vi "Update FP.vi"(6 "subpanel to main command event":T2, 7 "defer fp updates (T)":bool=TRUE, 8 "error in (no error)":errorcluster, 10 "fp refs":T1, 11 "steering frame ref in":refnum<data-value>) -> (0 "error out":errorcluster, 3 "steering frame ref out":refnum<data-value>)   [LabVIEW 2017, in "NI_Robotics_Configure Steering Frame.lvlib" / "Differential Frame Subpanel.lvlib"]
uses:
  <vilib>/robotics/Dialog/Configure Steering Frame/Differential Frame Subpanel/Differential Frame Subpanel.lvlib
  <vilib>/robotics/Steering/Differential Steering Frame/NI_Robotics_Differential Steering Frame.lvclass
  c:/Program Files (x86)/National Instruments/LabVIEW 2017/vi.lib/robotics/Steering/Steering Frame/NI_Robotics_Steering Frame.lvclass
  <vilib>/robotics/Dialog/Configure Steering Frame/Subpanel to Main Command Event.ctl
  <vilib>/robotics/Dialog/Configure Steering Frame/Subpanel to Main Command.ctl
  <vilib>/robotics/Dialog/Configure Steering Frame/Differential Frame Subpanel/FP Refs.ctl
  <vilib>/robotics/Steering/Differential Steering Frame/NI_Robotics_Differential Steering Frame.lvclass/NI_Robotics_Differential Steering Frame.ctl
  <vilib>/robotics/Steering/Steering Frame/NI_Robotics_Steering Frame.lvclass/NI_Robotics_Steering Frame.ctl
  <vilib>/robotics/Steering/Steering Frame/Get Single Wheel in Steering Frame.vi
  <vilib>/robotics/Steering/Steering Frame/Get Multiple Wheels in Steering Frame.vi
  <vilib>/robotics/Steering/Wheel/Get Fixed Wheel Information.vi
  <vilib>/robotics/Steering/Wheel/NI_Robotics_Wheel.lvclass
  <vilib>/robotics/Steering/Steering Frame/NI_Robotics_Steering Frame.lvclass
  c:/Program Files (x86)/National Instruments/LabVIEW 2017/vi.lib/robotics/Steering/Special Steering Frame/NI_Robotics_Special Steering Frame.lvclass
  <vilib>/robotics/Dialog/Configure Steering Frame/NI_Robotics_Configure Steering Frame.lvlib
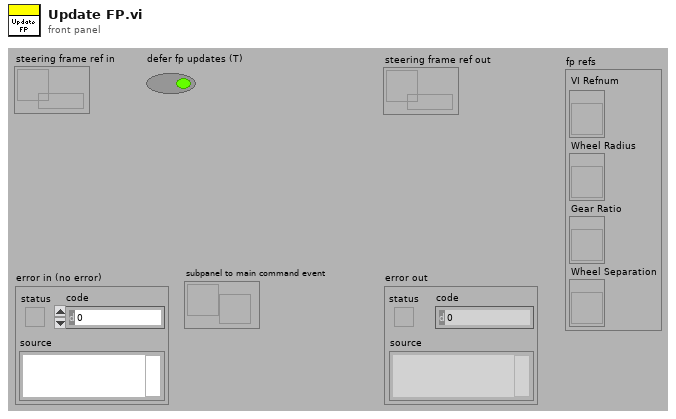
[diagram p1: front panel]
types:
  T1 = typedef "NI_Robotics_Configure Steering Frame.lvlib/Differential Frame Subpanel.lvlib/FP Refs.ctl" = cluster{"VI Refnum":refnum<vi>, "Wheel Radius":refnum<vi>, "Gear Ratio":refnum<vi>, "Wheel Separation":refnum<vi>}
  T2 = typedef "NI_Robotics_Configure Steering Frame.lvlib/Subpanel to Main Command Event.ctl" = refnum<user-event>
  T3 = typedef "NI_Robotics_Wheel.lvclass/Wheel Parameters.ctl" = cluster{"wheel radius":dbl, "gear ratio":dbl, "forward rotation direction":T4}
  T4 = typedef "NI_Robotics_Wheel.lvclass/Rotation Direction.ctl" = u16
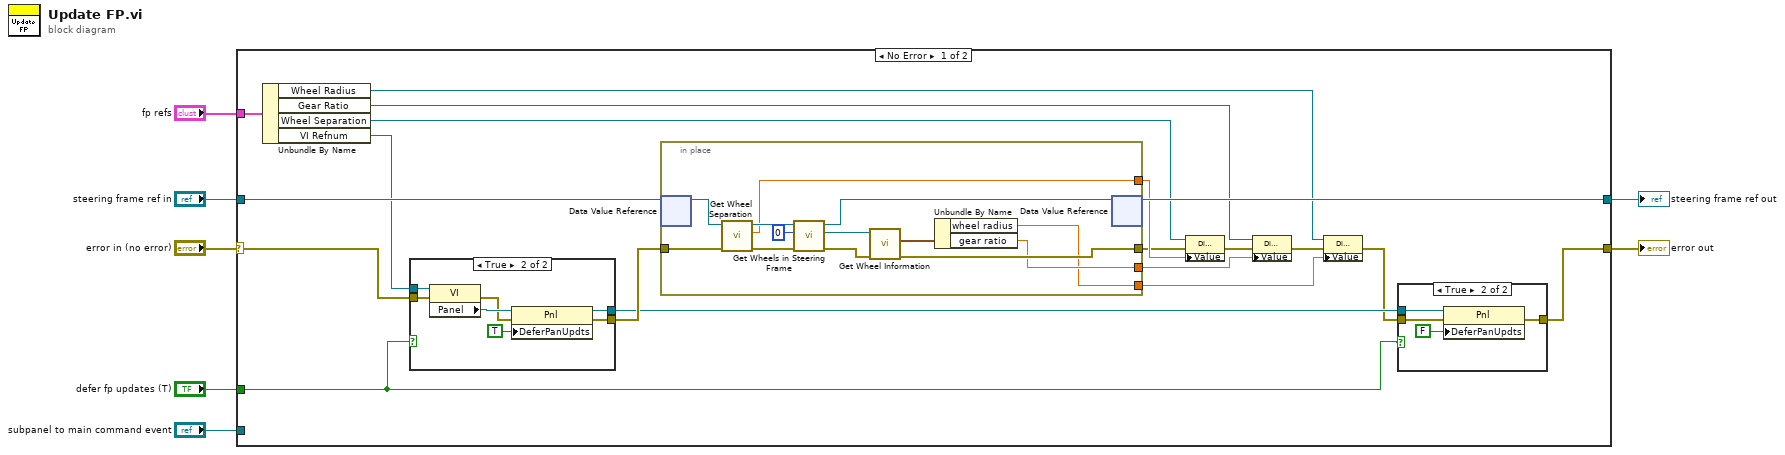
[diagram p0: block diagram]
diagram:
  n1 = case shown="No Error" "error in (no error)" {
    selector: "error in (no error)" -> [w22 w53]
    tunnel: "steering frame ref in" -> [w26 w54]
    tunnel: [w25 w54] -> w5
    tunnel: [w19 w53] -> w4
    tunnel: "subpanel to main command event" -> [_ _]
    tunnel: "fp refs" -> [w24 _]
    tunnel: "defer fp updates (T)" -> [w18 _]
    frame No Error {
      n2 = Unbundle By Name(w24) -> ("Wheel Radius"=w10:refnum<vi>, "Gear Ratio"=w12:refnum<vi>, "Wheel Separation"=w16:refnum<vi>, "VI Refnum"=w23:refnum<vi>)
      n3 = case shown="True" w18 {
        tunnel: [_ w37] -> w20
        tunnel: w23 -> [_ w36]
        tunnel: w22 -> [w32 w35]
        tunnel: [w32 w33] -> w21
        frame False {
        }
        frame True {
          n4 = property class="VI"(reference=w36, error in=w35) -> (error out=w34:errorcluster, "Panel"=w39:refnum<vi>)  [unwired: 1 out]
          n5 = property class="Pnl"(reference=w39, error in=w34, "DeferPanUpdts"=TRUE ("Defer Panel Updates")) -> (reference out=w37:refnum<vi>, error out=w33:errorcluster)
        }
      }
      n6 = in-place {
        in-place-border: w21 -> [w52]
        in-place-border: [w44] -> w15
        in-place-border: [w43] -> w17
        in-place-border: [w41] -> w11
        in-place-border: [w40] -> w9
        n7 = in-place-dvr #1(w26) -> (w51:refnum<class "NI_Robotics_Differential Steering Frame.lvclass">)  [unwired: 1 out]
        n8 = call <vilib>:"Get Wheel Separation.vi"("error in (no error)"=w52, "differential steering frame in"=w51) -> ("error out"=w50:errorcluster, "wheel separation"=w43:dbl, "differential steering frame out"=w49:refnum<class "NI_Robotics_Differential Steering Frame.lvclass">)  [unwired: 7 in]
        n9 = call-poly <vilib>:"Get Wheels in Steering Frame.vi"("error in (no error)"=w50, "wheel index"=0, "steering frame in"=w49) -> ("error out"=w45:errorcluster, "wheel"=w46:refnum<class "NI_Robotics_Wheel.lvclass">, "steering frame out"=w47:refnum<class "NI_Robotics_Differential Steering Frame.lvclass">)  [unwired: 2 in, 4 out]
        n10 = call-poly <vilib>:"Get Wheel Information.vi"("error in (no error)"=w45, "wheel in"=w46) -> ("error out"=w44:errorcluster, "wheel parameters"=w42:T3)  [unwired: 5 in, 3 out]
        n11 = Unbundle By Name(w42) -> ("wheel radius"=w40:dbl, "gear ratio"=w41:dbl)
        n12 = in-place-dvr #1(w47) -> (w25:refnum<data-value>)  [unwired: 1 out]
      }
      n13 = property class="DigNum (strict)"(reference=w16, error in=w15, "Value"=w17) -> (error out=w14:errorcluster)  [unwired: 1 out]
      n14 = property class="DigNum (strict)"(reference=w12, error in=w14, "Value"=w11) -> (error out=w13:errorcluster)  [unwired: 1 out]
      n15 = property class="DigNum (strict)"(reference=w10, error in=w13, "Value"=w9) -> (error out=w8:errorcluster)  [unwired: 1 out]
      n16 = case shown="True" w18 {
        tunnel: w20 -> [_ w30]
        tunnel: w8 -> [w27 w29]
        tunnel: [w27 w28] -> w19
        frame False {
        }
        frame True {
          n17 = property class="Pnl"(reference=w30, error in=w29, "DeferPanUpdts"=FALSE ("Defer Panel Updates")) -> (error out=w28:errorcluster)  [unwired: 1 out]
        }
      }
    }
    frame Error {
    }
  }
  "steering frame ref out" <- w5
  "error out" <- w4
